vi "Actuator Chart View.vi"(10 "User Events in":refnum<class "User Events.lvclass">) -> ()   [LabVIEW 2015, in "FAMT Views.lvlib"]
uses:
  FAMT Views.lvlib
  User Events/User Events.lvclass
  User Events/User Events.lvclass/User Events.ctl
  Typedefs/State Types.ctl
  Typedefs/Actuator Types.ctl
  Typedefs/FAMT Typedefs.lvlib
panel:
  out "Chart":T1(graph)
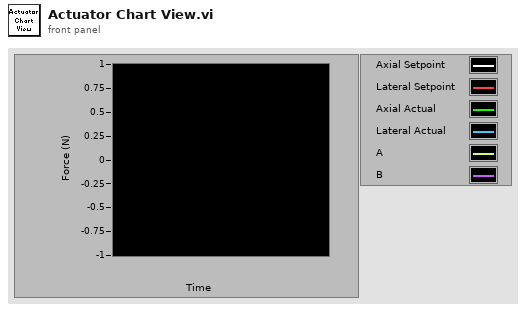
[diagram p1: front panel]
types:
  T1 = cluster{"Axial Demand":dbl, "Lateral Demand":dbl, dbl, dbl, dbl, dbl}
  T2 = typedef "FAMT Typedefs.lvlib/Publish Data Events.ctl" = cluster{"State":refnum<user-event>, "ErrorCode":refnum<user-event>, "FC1 ILC Outputs":refnum<user-event>, "LogPath":refnum<user-event>, "FC1 ILC Inputs":refnum<user-event>, "Scan Progress":refnum<user-event>, "FC2 ILC Outputs":refnum<user-event>, "FC2 ILC Inputs":refnum<user-event>}
  T3 = cluster{"Event Registration Refnum":refnum<event-registration>, "Event Registration Refnum":refnum<event-registration>}
  T4 = typedef "FAMT Typedefs.lvlib/State Types.ctl" = enum16{"Offline State", "Fault State", "Standby State", "Disabled State", "Enabled State", "Wait For User Input State", "Perform Scan State"}
  T5 = typedef "FAMT Typedefs.lvlib/Actuator Types.ctl" = enum16{"Single", "Dual", "Dual Outer"}
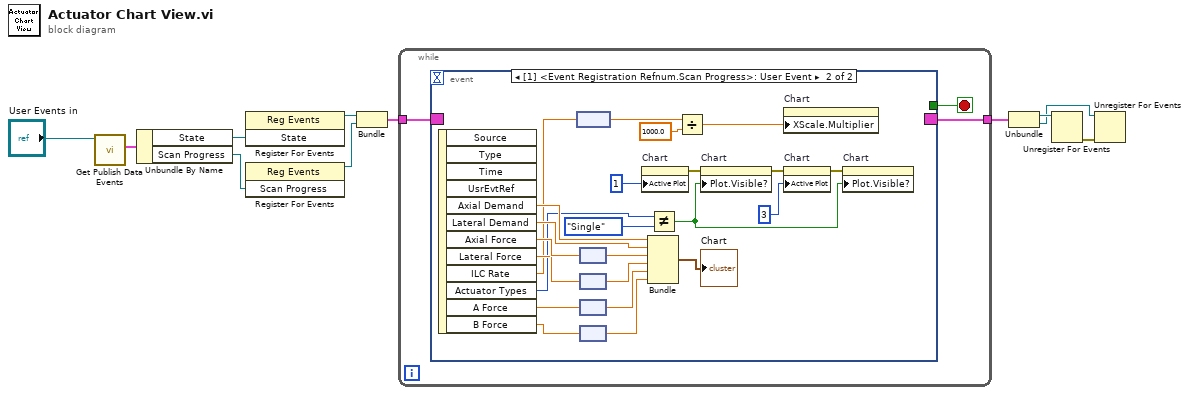
[diagram p0: block diagram]
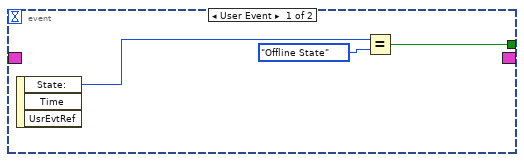
[diagram p2: hidden frame]
diagram:
  n1 = call "Get Publish Data Events.vi"("UserEvents in"="User Events in") -> ("Publish Data Events"=w8:T2)  [unwired: 9 in, 1 out]
  n2 = Unbundle By Name(w8) -> ("State"=w9:refnum<user-event>, "Scan Progress"=w7:refnum<user-event>)
  n3 = register-events(w9) -> (reference out=w11:refnum<event-registration>)  [unwired: 2 in, 1 out]
  n4 = register-events(w7) -> (reference out=w10:refnum<event-registration>)  [unwired: 2 in, 1 out]
  n5 = Bundle("Event Registration Refnum"=w11, "Event Registration Refnum"=w10) -> (w3:T3)  [unwired: 1 in]
  n6 = while {
    tunnel: w3 -> [w14]
    tunnel: [w13] -> w2
    stop <- w12 stop-if-true
    n7 = event shown="[1] <Event Registration Refnum.Scan Progress>: User Event" {
      selector: w14 -> [_ _]
      dyn-events: [_ _] -> w13
      timeout: _ -> [_ _]
      tunnel: [w16 _] -> w12
      event User Event {
        n8 = event-data() -> ("State:"=w15:T4)  [unwired: 1 in, 2 out]
        n9 = Equal?(x=w15, y=State_Types."Offline State") -> (x = y?=w16:bool)
      }
      event User Event {
        n10 = event-data() -> ("Axial Demand"=w37:dbl, "Lateral Demand"=w31:dbl, "Axial Force"=w36:dbl[unit], "Lateral Force"=w33:dbl[unit], "ILC Rate"=w30:dbl[unit], "Actuator Types"=w29:T5, "A Force"=w21:dbl[unit], "B Force"=w20:dbl[unit])  [unwired: 1 in, 4 out]
        n11 = node(w30) -> (w39:dbl)
        n12 = node(w36) -> (w35:dbl)
        n13 = node(w33) -> (w34:dbl)
        n14 = node(w21) -> (w19:dbl)
        n15 = node(w20) -> (w18:dbl)
        n16 = property on="Chart" class="WFChart (strict)"("Active Plot"=u32 1) -> (error out=w26:errorcluster)  [unwired: 2 in, 1 out]
        n17 = Bundle("Axial Demand"=w37, "Lateral Demand"=w31, w35, w34, w19, w18) -> (→"Chart":T1)  [unwired: 1 in]
        n18 = Not Equal?(x=w29, y=Actuator_Types."Single") -> (x != y?=w27:bool)
        n19 = Divide(x=w39, y=1000.0) -> (x/y=w38:dbl)
        n20 = property on="Chart" class="WFChart (strict)"(error in=w26, "Plot.Visible?"=w27) -> (error out=w25:errorcluster)  [unwired: 1 in, 1 out]
        n21 = property on="Chart" class="WFChart (strict)"("XScale.Multiplier"=w38) -> ()  [unwired: 2 in, 2 out]
        n22 = property on="Chart" class="WFChart (strict)"(error in=w25, "Active Plot"=u32 3) -> (error out=w24:errorcluster)  [unwired: 1 in, 1 out]
        n23 = property on="Chart" class="WFChart (strict)"(error in=w24, "Plot.Visible?"=w27) -> ()  [unwired: 1 in, 2 out]
      }
    }
  }
  n24 = Unbundle(w2) -> ("Event Registration Refnum"=w6:refnum<event-registration>, "Event Registration Refnum"=w5:refnum<event-registration>)
  n25 = Unregister For Events(event registration refnum=w6) -> (error out=w4:errorcluster)  [unwired: 1 in]
  n26 = Unregister For Events(event registration refnum=w5, error in=w4) -> ()  [unwired: 1 out]
